vi "test presicion.vi"() -> ()   [LabVIEW 2019]
panel:
  in  "array":cluster{"x":dbl[], "y":dbl[]}[](array[cluster])
  out "Array":dbl[](array[numeric])=[1.11, 1.11, 1.11, 1.11, 1.11, 1.11]
  in  "cluster":cluster{"x":dbl[], "y":dbl[]}
  in  "Numeric":dbl format="%#.13f"
  out "XY":cluster{"Array out":dbl[], "Array out":dbl[]}[](graph)
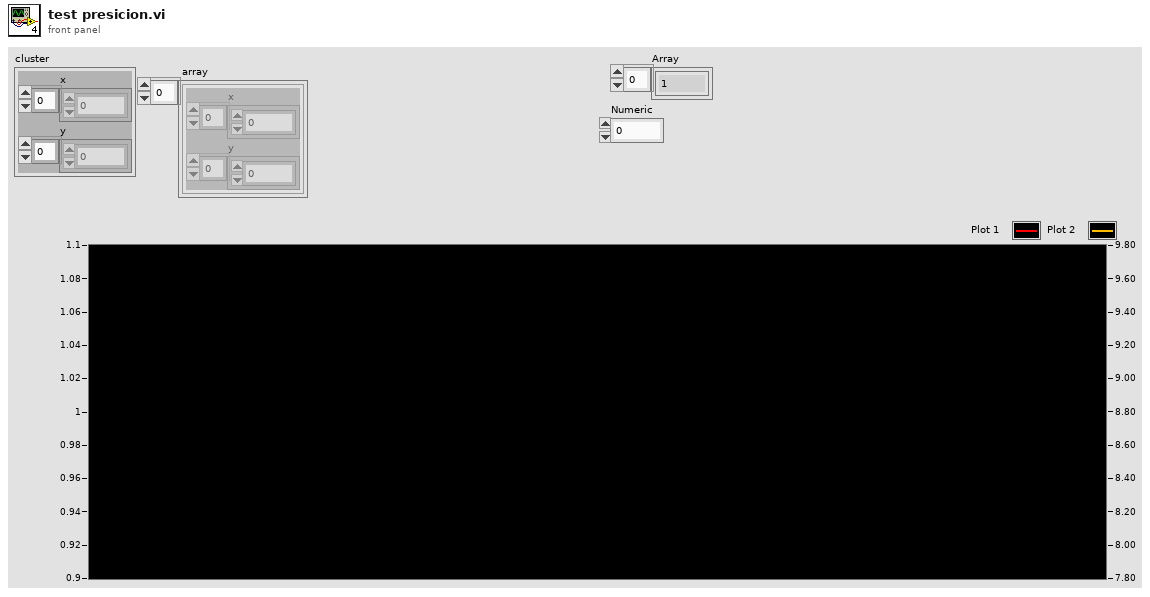
[diagram p1: front panel]
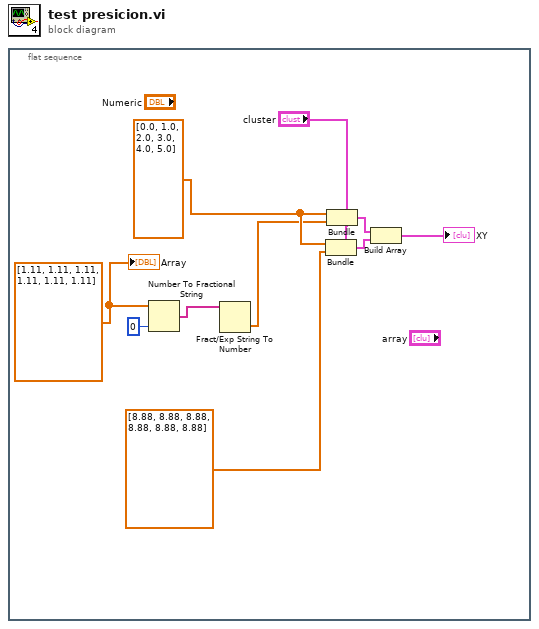
[diagram p0: block diagram]
diagram:
  n1 = flat-sequence {
    frame #0 {
      w4 = dbl[] [1.11, 1.11, 1.11, 1.11, 1.11, 1.11]
      w7 = dbl[] [0.0, 1.0, 2.0, 3.0, 4.0, 5.0]
      n2 = Number To Fractional String(number=w4, precision (6)=i16 0) -> (F-format string=w2:string[])  [unwired: 2 in]
      n3 = Fract/Exp String To Number(string=w2) -> (number=w1:dbl[])  [unwired: 3 in, 1 out]
      n4 = Bundle(cluster="cluster", "x"=w7, "y"=dbl[] [8.88, 8.88, 8.88, 8.88, 8.88, 8.88]) -> (w9:cluster{"x":dbl[], "y":dbl[]})
      n5 = Bundle(cluster="cluster", "x"=w7, "y"=w1) -> (w10:cluster{"x":dbl[], "y":dbl[]})
      n6 = Build Array(w10, w9) -> (→"XY":cluster{"x":dbl[], "y":dbl[]}[])
      "Array" <- w4
    }
  }
